vi "pl1000SetTrigger.vi"(0 "pl1000 handle":i16, 1 "dir":enum16{"rising edge", "falling edge"}(ring), 2 "autoMs":u16, 5 "enabled":bool, 7 "autoTrigger":bool, 9 "channel":u16, 11 "error in (no error)":errorcluster, 12 "threshold":u16, 13 "hysteresis":u16, 14 "delay":dbl) -> (4 "pl1000 handle out":i16, 15 "error out":errorcluster)   [LabVIEW 2016, in "pl1000.lvlib"]
doc: "This function sets up the trigger, which controls when the unit starts capturing data\n\nenabled: whether to enable or disable the trigger:\n\nauto_trigger: whether or not to re-arm the trigger automatically after each trigger event:\n\nauto_ms: time in milliseconds after which the unit will auto-trigger if the trigger condition is not met\n\nchannel: which channel to trigger on\n\ndir: which edge to trigger on\n\nthreshold: trigger threshold (the level at which the trigger will activate) in ADC counts\n\nhysteresis: trigger hysteresis in ADC counts. This is the difference between the upper and lower thresholds. The signal must then pass through both thresholds in the same direction in order to activate the trigger, so that there are fewer unwanted trigger events caused by noise. The minimum value allowed is 1. \n\ndelay: delay between the trigger event and the start of the block as a percentage of the block size. 0% means that the trigger event is the first data value in the block, and -50% means that the trigger event is in the middle of the block."
uses:
  pl1000.lvlib
  pl1000.dll
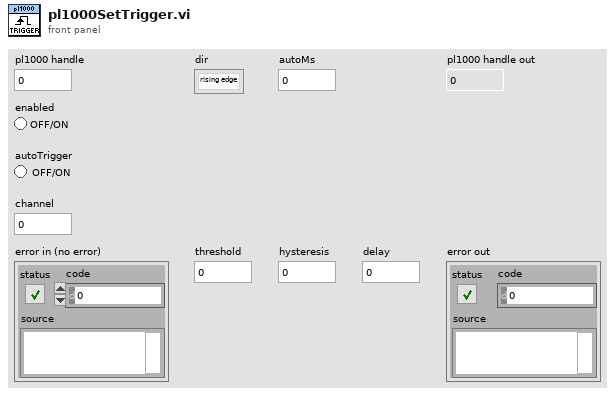
[diagram p1: front panel]
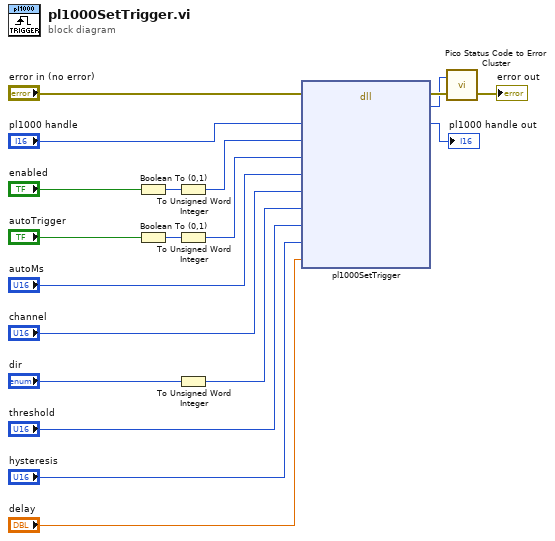
[diagram p0: block diagram]
diagram:
  n1 = Boolean To (0,1)(Boolean="enabled") -> (0, 1=w12:i16)
  n2 = Boolean To (0,1)(Boolean="autoTrigger") -> (0, 1=w10:i16)
  n3 = To Unsigned Word Integer(number=w12) -> (unsigned 16bit integer=w11:u16)
  n4 = To Unsigned Word Integer(number=w10) -> (unsigned 16bit integer=w8:u16)
  n5 = To Unsigned Word Integer(number="dir") -> (unsigned 16bit integer=w4:u16)
  n6 = dll-call lib="pl1000.dll" fn="pl1000SetTrigger"(error in="error in (no error)", "handle"="pl1000 handle", "enabled"=w11, "autoTrigger"=w8, "autoMs"="autoMs", "channel"="channel", "dir"=w4, "threshold"="threshold", "hysteresis"="hysteresis", "delay"="delay") -> (error out=w17:errorcluster, "status"=w16:u32, "handle"=→"pl1000 handle out":i16)  [unwired: 10 in, 1 out]
  n7 = call "Pico Status Code to Error Cluster.vi"("error in"=w17, "PICO_STATUS"=w16) -> ("error out"=→"error out":errorcluster)  [unwired: 1 in]
